vi "Data Format.vi"(7 "Mode (T: Set)":bool=TRUE, 8 "Error In (no error)":errorcluster, 9 "Order  (0: Normal)":u16(ring) items=["Normal", "Swapped"], 10 "Source (0: Real 32)":u16(ring) items=["Real 32", "Real 64", "ASCII"], 11 "VISA Resource Name":refnum<visa-resource-name>) -> (0 "Error Out":errorcluster, 2 "Source":u16(ring) items=["Real 32", "Real 64", "ASCII"], 3 "VISA Resource Name Out":refnum<visa-resource-name>)   [LabVIEW 2018, in "Agilent PNA Series.lvlib"]
doc: "This VI set the data format for transfer and order of transferred bytes."
uses:
  Agilent PNA Series.lvlib
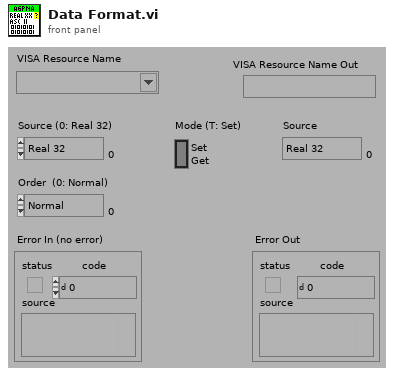
[diagram p1: front panel]
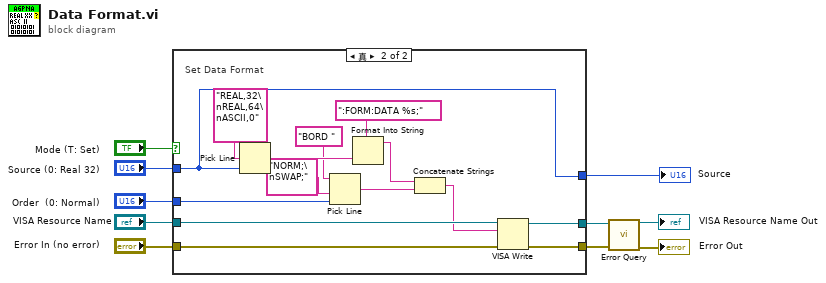
[diagram p0: block diagram]
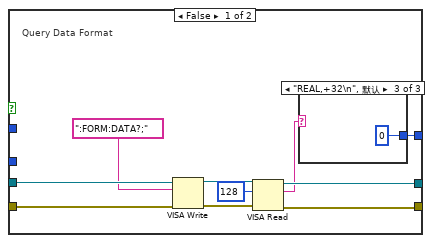
[diagram p2: hidden frame]
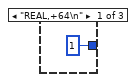
[diagram p3: hidden frame]
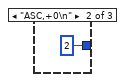
[diagram p4: hidden frame]
diagram:
  n1 = case shown="真" "Mode (T: Set)" {
    tunnel: "VISA Resource Name" -> [w20 w37]
    tunnel: "Error In (no error)" -> [w19 w36]
    tunnel: [w16 w32] -> w4
    tunnel: [w15 w31] -> w3
    tunnel: "Source (0: Real 32)" -> [_ w24]
    tunnel: "Order  (0: Normal)" -> [_ w28]
    tunnel: [w12 w24] -> w5
    frame False {
      # "Query Data Format"
      n2 = VISA Write(VISA resource name=w20, write buffer=":FORM:DATA?;" ("format string"), error in (no error)=w19) -> (VISA resource name out=w18:refnum<visa-resource-name>, error out=w17:errorcluster)  [unwired: 1 out]
      n3 = VISA Read(VISA resource name=w18, byte count=u32 128 ("byte count (0)"), error in (no error)=w17) -> (VISA resource name out=w16:refnum<visa-resource-name>, read buffer=w13:string, error out=w15:errorcluster)  [unwired: 1 out]
      n4 = case shown="\"REAL,+32\\n\", 默认" w13 {
        tunnel: [1 2 0] -> w12
        frame "REAL,+64\n" {
        }
        frame "ASC,+0\n" {
        }
        frame "REAL,+32\n", Default {
        }
      }
    }
    frame True {
      # "Set Data Format"
      n5 = Pick Line(multi-line string="REAL,32\nREAL,64\nASCII,0" ("string (\"\")"), line index=w24) -> (output string=w33:string)  [unwired: 1 in]
      n6 = Pick Line(string ("")="BORD ", multi-line string="NORM;\nSWAP;" ("string (\"\")"), line index=w28) -> (output string=w26:string)
      n7 = Format Into String(format string=":FORM:DATA %s;", w33) -> (resulting string=w27:string)  [unwired: 2 in, 1 out]
      n8 = Concatenate Strings(w27, w26) -> (w35:string)
      n9 = VISA Write(VISA resource name=w37, write buffer=w35, error in (no error)=w36) -> (VISA resource name out=w32:refnum<visa-resource-name>, error out=w31:errorcluster)  [unwired: 1 out]
    }
  }
  "Source" <- w5
  n10 = call "Error Query.vi"("VISA Resource Name"=w4, "error in (no error)"=w3) -> ("VISA Resource Name Out"=→"VISA Resource Name Out":refnum<visa-resource-name>, "error out"=→"Error Out":errorcluster)  [unwired: 10 in, 2 out]
